vi "To String.vi"(8 "error in (no error)":errorcluster, 11 "Raw Message in":refnum<class "Raw Message.lvclass">) -> (0 "error out":errorcluster, 2 "String Representation":string, 3 "Raw Message out":refnum<class "Raw Message.lvclass">)   [LabVIEW 2020, in "Protobuf RAW.lvlib" / "Raw Message.lvclass"]
uses:
  Message/Raw Message.lvclass
  Message/Raw Message.lvclass/Raw Message.ctl
  String Representable/String Representable.lvclass
  Message/Read Tags.vi
  Tag/Basic Type.lvclass
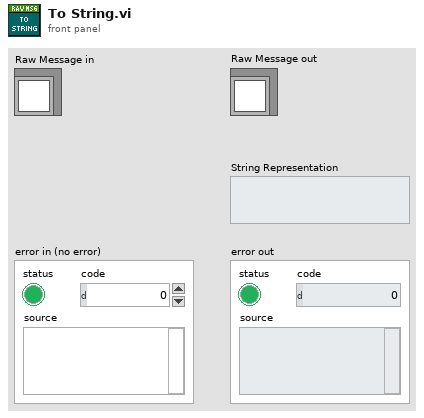
[diagram p1: front panel]
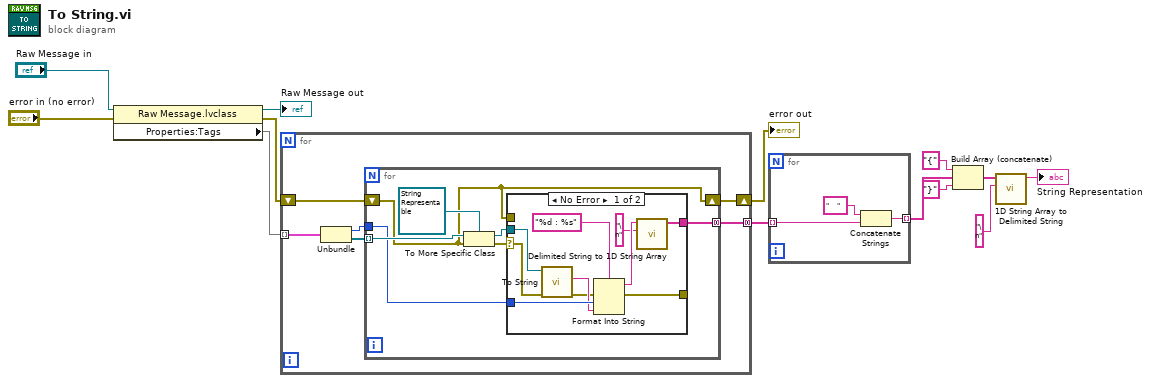
[diagram p0: block diagram]
diagram:
  n1 = property class="Raw Message.lvclass"(reference="Raw Message in", error in="error in (no error)") -> (reference out=→"Raw Message out":refnum<class "Raw Message.lvclass">, error out=w10:errorcluster, "Properties:Tags"=w9:map{u32, refnum<class "Basic Type.lvclass">[]})
  n2 = for {
    tunnel: w9 -> [w19] mode=indexing
    tunnel: [w16] -> w5 mode=concatenating
    shift-right: [w14] -> w6
    shift-left: w10 -> [w15]
    n3 = Unbundle(w19) -> ("ID"=w18:u32, "Tag"=w17:refnum<class "Basic Type.lvclass">[])
    n4 = for {
      tunnel: w18 -> [w24]
      tunnel: w17 -> [w26] mode=indexing
      tunnel: [w23] -> w16 mode=concatenating
      shift-right: [w20] -> w14
      shift-left: w15 -> [w20]
      n5 = To More Specific Class(target class=refnum<class "String Representable.lvclass"> refnum ("Protobuf Encode.lvlib:String Representable.lvclass"), reference=w26, error in=w20) -> (specific class reference=w25:refnum<class "String Representable.lvclass">, error out=w22:errorcluster)
      n6 = case shown="No Error" w22 {
        selector: w22 -> [w32 _]
        tunnel: w25 -> [w33 _]
        tunnel: w24 -> [w35 _]
        tunnel: [w27 _] -> w23
        tunnel: [w34 w37] -> _
        tunnel: w20 -> [_ w37]
        frame No Error {
          n7 = call-dynamic "To String.vi"("error in (no error)"=w32, "String Representable in"=w33) -> ("error out"=w30:errorcluster, "String"=w31:string)  [unwired: 7 in, 1 out]
          n8 = Format Into String(format string="%d : %s", error in=w30, w35, w31) -> (resulting string=w29:string, error out=w34:errorcluster)  [unwired: 1 in]
          n9 = call <vilib>:"Delimited String to 1D String Array.vi"("delimiter"="\n", "delimited string"=w29) -> ("string array"=w27:string[])  [unwired: 9 in]
        }
        frame Error {
        }
      }
    }
  }
  "error out" <- w6
  n10 = for {
    tunnel: w5 -> [w40] mode=indexing
    tunnel: [w39] -> w4 mode=indexing
    n11 = Concatenate Strings("    " ("string"), w40) -> (w39:string)
  }
  n12 = Build Array (concatenate)("{", w4, "}") -> (w3:string[])
  n13 = call <vilib>:"1D String Array to Delimited String.vi"("delimiter"="\n", "string array"=w3) -> ("delimited string"=→"String Representation":string)  [unwired: 9 in]
